vi "))Channel.vi"(0 "channel in":T1, 1 "This VI":refnum<vi>, 5 "subchannel":i32, 7 "channelOp":T4, 9 "params":T3={"last element in"=FALSE, "valid"=FALSE, "abort in"=FALSE, "event priority (norm)"=enum."normal priority"}, 11 "element in":cluster{"cmd":string, "data":variant}, 12 "# event structures":u16=2) -> (3 "last element out":bool, 4 "channel out":T1, 6 "event registration refnums":refnum<event-registration>[](array[refnum]), 8 "This VI out":refnum<vi>, 14 "aborted?":bool)   [LabVIEW 2019, in "Event MessengerM.lvlib"]
uses:
  Event MessengerM.lvlib
  Instantiate.vi
  EventMessengerMData.lvclass
  ChannelOp.ctl
  <vilib>/event_ctls.llb/usereventprio.ctl
  ))Channel.ctl
  Event Data.ctl
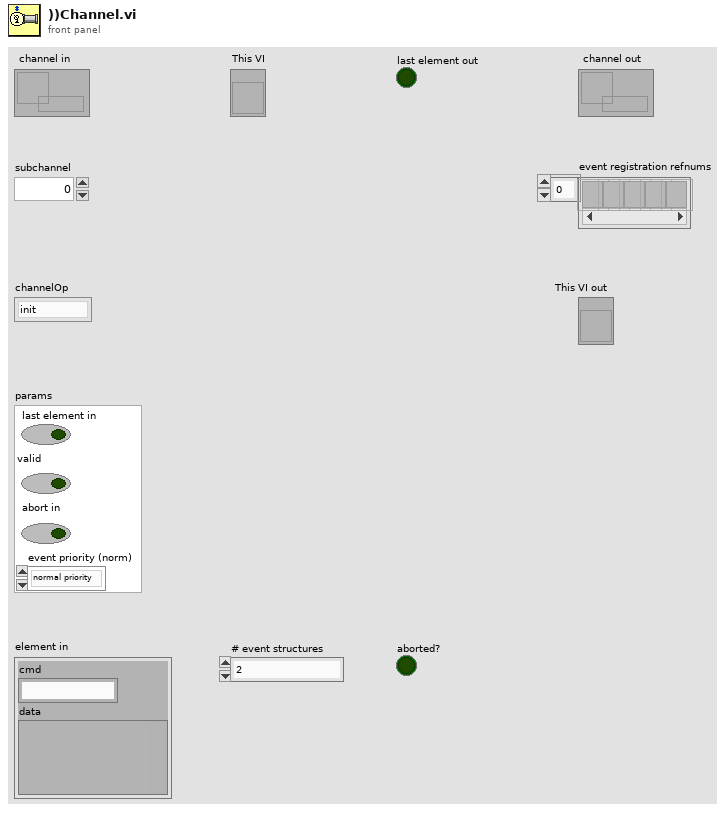
[diagram p1: front panel]
types:
  T1 = typedef "Event MessengerM.lvlib/))Channel.ctl" = refnum<queue>
  T2 = typedef "usereventprio.ctl" = enum32{"high priority", "normal priority"}
  T3 = cluster{"last element in":bool, "valid":bool, "abort in":bool, "event priority (norm)":T2}
  T4 = typedef "Event MessengerM.lvlib/ChannelOp.ctl" = enum16{"init", "write", "register", "replicate", "probe"}
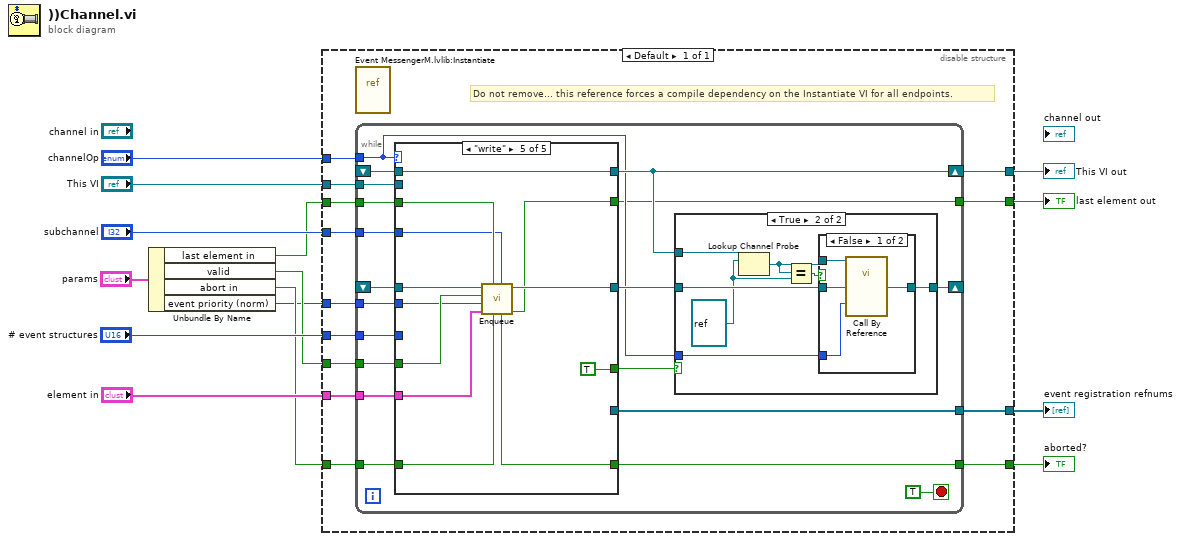
[diagram p0: block diagram]
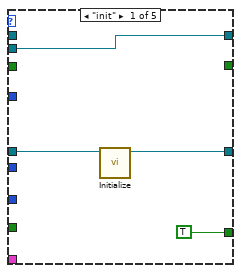
[diagram p4: hidden frame]
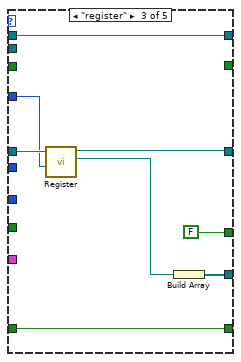
[diagram p6: hidden frame]
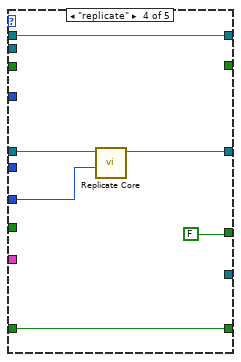
[diagram p7: hidden frame]
diagram:
  n1 = Unbundle By Name("params") -> ("last element in"=w4:bool, "valid"=w3:bool, "abort in"=w2:bool, "event priority (norm)"=w1:T2)
  n2 = disable-structure shown="Default" {
    disable-tunnel: "element in" -> [w22]
    disable-tunnel: "This VI" -> [w27]
    disable-tunnel: [w26] -> w13
    disable-tunnel: "channelOp" -> [w25]
    disable-tunnel: [w24] -> w11
    disable-tunnel: "subchannel" -> [w23]
    disable-tunnel: [w21] -> w9
    disable-tunnel: w2 -> [w20]
    disable-tunnel: [w19] -> w8
    disable-tunnel: w4 -> [w18]
    disable-tunnel: w3 -> [w17]
    disable-tunnel: w1 -> [w16]
    disable-tunnel: "# event structures" -> [w15]
    frame Enabled {
      # "Do not remove... this reference forces a compile dependency on the Instantiate VI for all endpoints."
      n3 = vi-ref "Event MessengerM.lvlib:Instantiate.vi"() -> ()  [unwired: 1 out]
      n4 = while {
        tunnel: w25 -> [w38]
        shift-right: [w40] -> _
        shift-left: _ -> [w45]
        tunnel: w27 -> [w44]
        shift-right: [w42] -> w26
        shift-left: _ -> [w43]
        tunnel: [w37] -> w24
        tunnel: w23 -> [w36]
        tunnel: w22 -> [w35]
        tunnel: [w34] -> w21
        tunnel: w20 -> [w33]
        tunnel: [w32] -> w19
        tunnel: w18 -> [w31]
        tunnel: w17 -> [w30]
        tunnel: w16 -> [w29]
        tunnel: w15 -> [w28]
        stop <- TRUE stop-if-true
        n5 = case shown="\"write\"" w38 {
          tunnel: w45 -> [w60 w64 w72 w77 w90]
          tunnel: [w62 w64 w71 w78 w89] -> w41
          tunnel: w35 -> [_ _ _ _ w84]
          tunnel: [TRUE _ FALSE ("wait") FALSE ("wait") TRUE ("not an occurrence?")] -> w39
          tunnel: w44 -> [w63 _ _ _ _]
          tunnel: [w63 w65 w73 w79 w91] -> w42
          tunnel: w43 -> [_ w65 w73 w79 w91]
          tunnel: [_ _ w69 _ _] -> w37
          tunnel: w36 -> [_ _ w68 _ w83]
          tunnel: [_ _ w66 w74 w88] -> w34
          tunnel: w33 -> [_ _ w66 w74 w87]
          tunnel: [_ _ _ _ w86] -> w32
          tunnel: w31 -> [_ _ _ _ w85]
          tunnel: w30 -> [_ _ _ _ w82]
          tunnel: w29 -> [_ _ _ _ w81]
          tunnel: w28 -> [_ _ _ w76 _]
          frame "init" {
            n6 = call "Initialize.vi"("data in"=w60) -> ("data out"=w62:refnum<class "EventMessengerMData.lvclass">)  [unwired: 9 in, 1 out]
          }
          frame "probe" {
            # "Probe case only exists to get the This VI Out."
          }
          frame "register" {
            n7 = call "Register.vi"("subchannel"=w68, "data in"=w72) -> ("event registration refnum"=w70:refnum<event-registration>, "data out"=w71:refnum<class "EventMessengerMData.lvclass">)  [unwired: 8 in]
            n8 = Build Array(w70) -> (w69:refnum<event-registration>[])
          }
          frame "replicate" {
            n9 = call "Replicate Core.vi"("# event structures"=w76, "data in"=w77) -> ("data out"=w78:refnum<class "EventMessengerMData.lvclass">)  [unwired: 8 in, 1 out]
          }
          frame "write" {
            n10 = call "Enqueue.vi"("subchannel"=w83, "abort? (F)"=w87, "last element? (F)"=w85, "element"=w84, "event priority"=w81, "is valid? (T)"=w82, "data in"=w90) -> ("last element?"=w86:bool, "data out"=w89:refnum<class "EventMessengerMData.lvclass">, "aborted?"=w88:bool)  [unwired: 2 in]
          }
        }
        n11 = case shown="True" w39 {
          tunnel: w42 -> [_ w54]
          tunnel: w41 -> [w47 w53]
          tunnel: [w47 w52] -> w40
          tunnel: w38 -> [_ w48]
          frame False {
          }
          frame True {
            w49 = refnum<vi> refnum ("This VI")
            n12 = Lookup Channel Probe(0:w54, 1:w49) -> (9:w50:refnum<vi>)  [unwired: 1 in, 1 out]
            n13 = Equal?(x=w50, y=w49) -> (x = y?=w51:bool)
            n14 = case shown="False" w51 {
              tunnel: w50 -> [w58 _]
              tunnel: w53 -> [w57 w59]
              tunnel: [w56 w59] -> w52
              tunnel: w48 -> [w55 _]
              frame False {
                n15 = call-by-ref "?"(reference=w58, "channelOp"=w55, "EventMessengerMData"=w57) -> ("EventMessengerMData"=w56:refnum<class "EventMessengerMData.lvclass">)  [unwired: 2 in, 2 out]
              }
              frame True {
              }
            }
          }
        }
      }
    }
  }
  "This VI out" <- w13
  "event registration refnums" <- w11
  "aborted?" <- w9
  "last element out" <- w8
